vi "Optim joy manipulator.vi"(8 "device index":i32=7, 11 "wyszukaj xbox":bool) -> (0 "error out":errorcluster, 1 "Refnum out":refnum<k1>, 2 "output cluster":T1, 3 "axis info":T4, 5 "wysylanie":bool, 7 "change arm mode":bool)   [LabVIEW 2015]
uses:
  wyj manip.ctl
  <vilib>/Utility/inputDevices.llb/joystickAcquire.vi
  <vilib>/MakerHub/Xbox-One-Controller/LMH-Xbox-One-Controller.lvlib
panel:
  out "direction info":T2
  out "button info":T3
  out "Cluster":T5
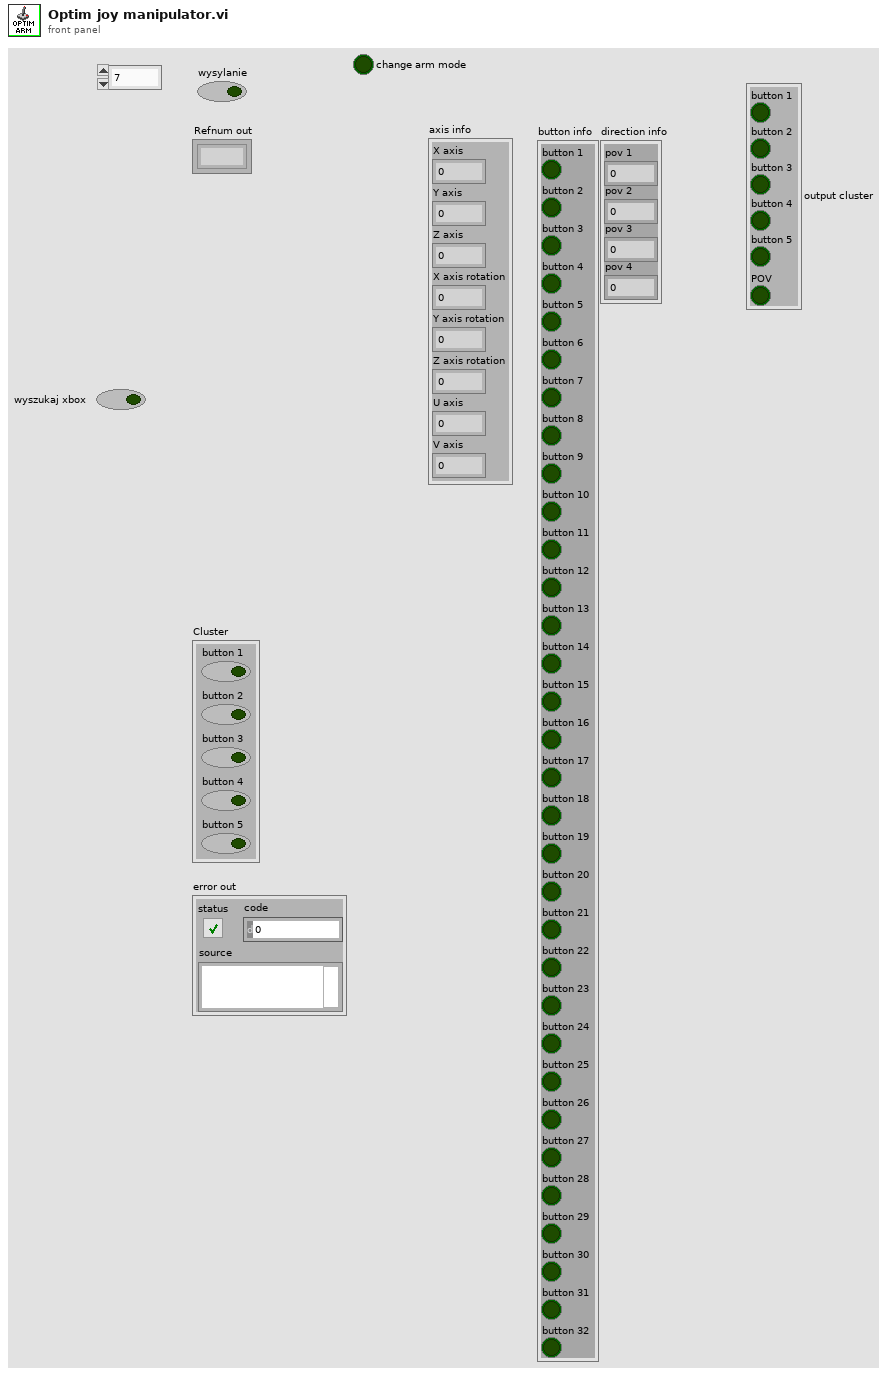
[diagram p1: front panel]
types:
  T1 = typedef "wyj manip.ctl" = cluster{"button 1":bool, "button 2":bool, "button 3":bool, "button 4":bool, "button 5":bool, "POV":bool}
  T2 = cluster{"pov 1":i32, "pov 2":i32, "pov 3":i32, "pov 4":i32}
  T3 = cluster{"button 1":bool, "button 2":bool, "button 3":bool, "button 4":bool, "button 5":bool, "button 6":bool, "button 7":bool, "button 8":bool, "button 9":bool, "button 10":bool, "button 11":bool, "button 12":bool, "button 13":bool, "button 14":bool, "button 15":bool, "button 16":bool, "button 17":bool, "button 18":bool, "button 19":bool, "button 20":bool, "button 21":bool, "button 22":bool, "button 23":bool, "button 24":bool, "button 25":bool, "button 26":bool, "button 27":bool, "button 28":bool, "button 29":bool, "button 30":bool, "button 31":bool, "button 32":bool}
  T4 = cluster{"X axis":i32, "Y axis":i32, "Z axis":i32, "X axis rotation":i32, "Y axis rotation":i32, "Z axis rotation":i32, "U axis":i32, "V axis":i32}
  T5 = cluster{"button 1":bool, "button 2":bool, "button 3":bool, "button 4":bool, "button 5":bool}
  T6 = typedef "LMH-Xbox-One-Controller.lvlib/Xbox Controller Device.ctl" = cluster{"Device Index":i32, "Device Name":string}
  T7 = cluster{"button 1":bool, "button 2":bool, "button 3":bool, "button 4":bool, "button 5":bool, bool}
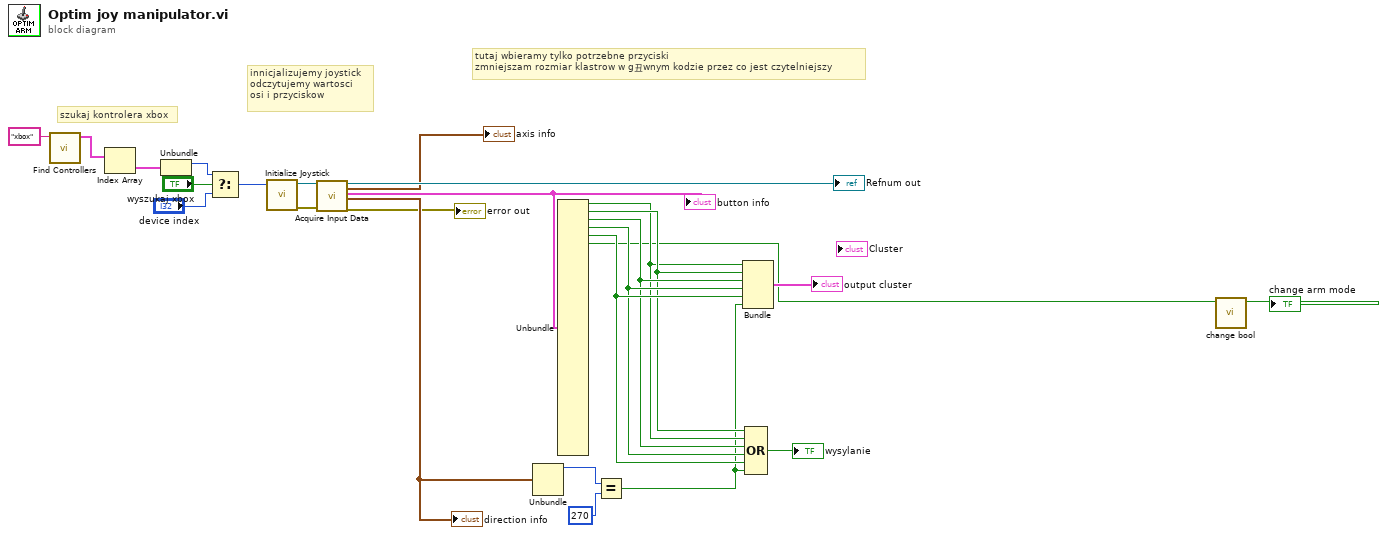
[diagram p0: block diagram]
diagram:
  # "szukaj kontrolera xbox"
  # "innicjalizujemy joystick\nodczytujemy wartosci \nosi i przyciskow"
  # "tutaj wbieramy tylko potrzebne przyciski \nzmniejszam rozmiar klastrow w g丑wnym kodzie przez co jest czytelniejszy"
  n1 = call <vilib>:"Find Controllers.vi"("name"="xbox" ("search string/char (-)")) -> ("Controllers"=w9:T6[])  [unwired: 9 in, 1 out]
  n2 = Index Array(array=w9) -> (element=w8:T6)  [unwired: 1 in]
  n3 = Unbundle(w8) -> ("Device Index"=w5:i32)  [unwired: 1 out]
  n4 = Select(t=w5, s="wyszukaj xbox", f="device index") -> (s? t:f=w7:i32)
  n5 = call <vilib>:"Initialize Joystick.vi"("device index"=w7) -> ("error out"=w19:errorcluster, "device ID"=w12:refnum<k1>)  [unwired: 9 in]
  n6 = call-poly <vilib>:"Acquire Input Data.vi"("device ID"=w12, "error in (no error)"=w19) -> ("device ID"=→"Refnum out":refnum<k1>, "axis info"=→"axis info":T4, "button info"=w14:T3, "direction info"=w20:T2, "error out"=→"error out":errorcluster)  [unwired: 13 in]
  "button info" <- w14
  "direction info" <- w20
  n7 = Unbundle(w20) -> ("pov 1"=w15:i32)  [unwired: 3 out]
  n8 = Unbundle(w14) -> ("button 1"=w22:bool, "button 2"=w23:bool, "button 3"=w24:bool, "button 4"=w25:bool, "button 5"=w26:bool, "button 6"=w2:bool)  [unwired: 26 out]
  n9 = Equal?(x=w15, y=270) -> (x = y?=w11:bool)
  n10 = Bundle("button 1"=w22, "button 2"=w23, "button 3"=w24, "button 4"=w25, "button 5"=w26, w11) -> (→"output cluster":T7)  [unwired: 1 in]
  n11 = Compound Arithmetic op=OR(w23, w22, w24, w25, w26, w11) -> (→"wysylanie":bool)
  n12 = call "change bool.vi"("button 6"=w2) -> ("change arm mode"=→"change arm mode":bool)  [unwired: 10 in]
